vi "query.vi"(0 "object in":refnum<class "sqlite.lvclass">, 1 "database":string(combo), 2 "table输入":string(combo), 3 "columns":string[](array[string]), 4 "condition":string, 5 "error in (no error)":errorcluster) -> (14 "object out":refnum<class "sqlite.lvclass">, 15 "data":string[][](table), 16 "columns输出":string[](array[string]), 17 "拆分数据":bool, 19 "error out":errorcluster)   [LabVIEW 2016, in "sqlite.lvclass"]
uses:
  sqlite.lvclass
  <vilib>/Utility/sysdir.llb/System Directory Type.ctl
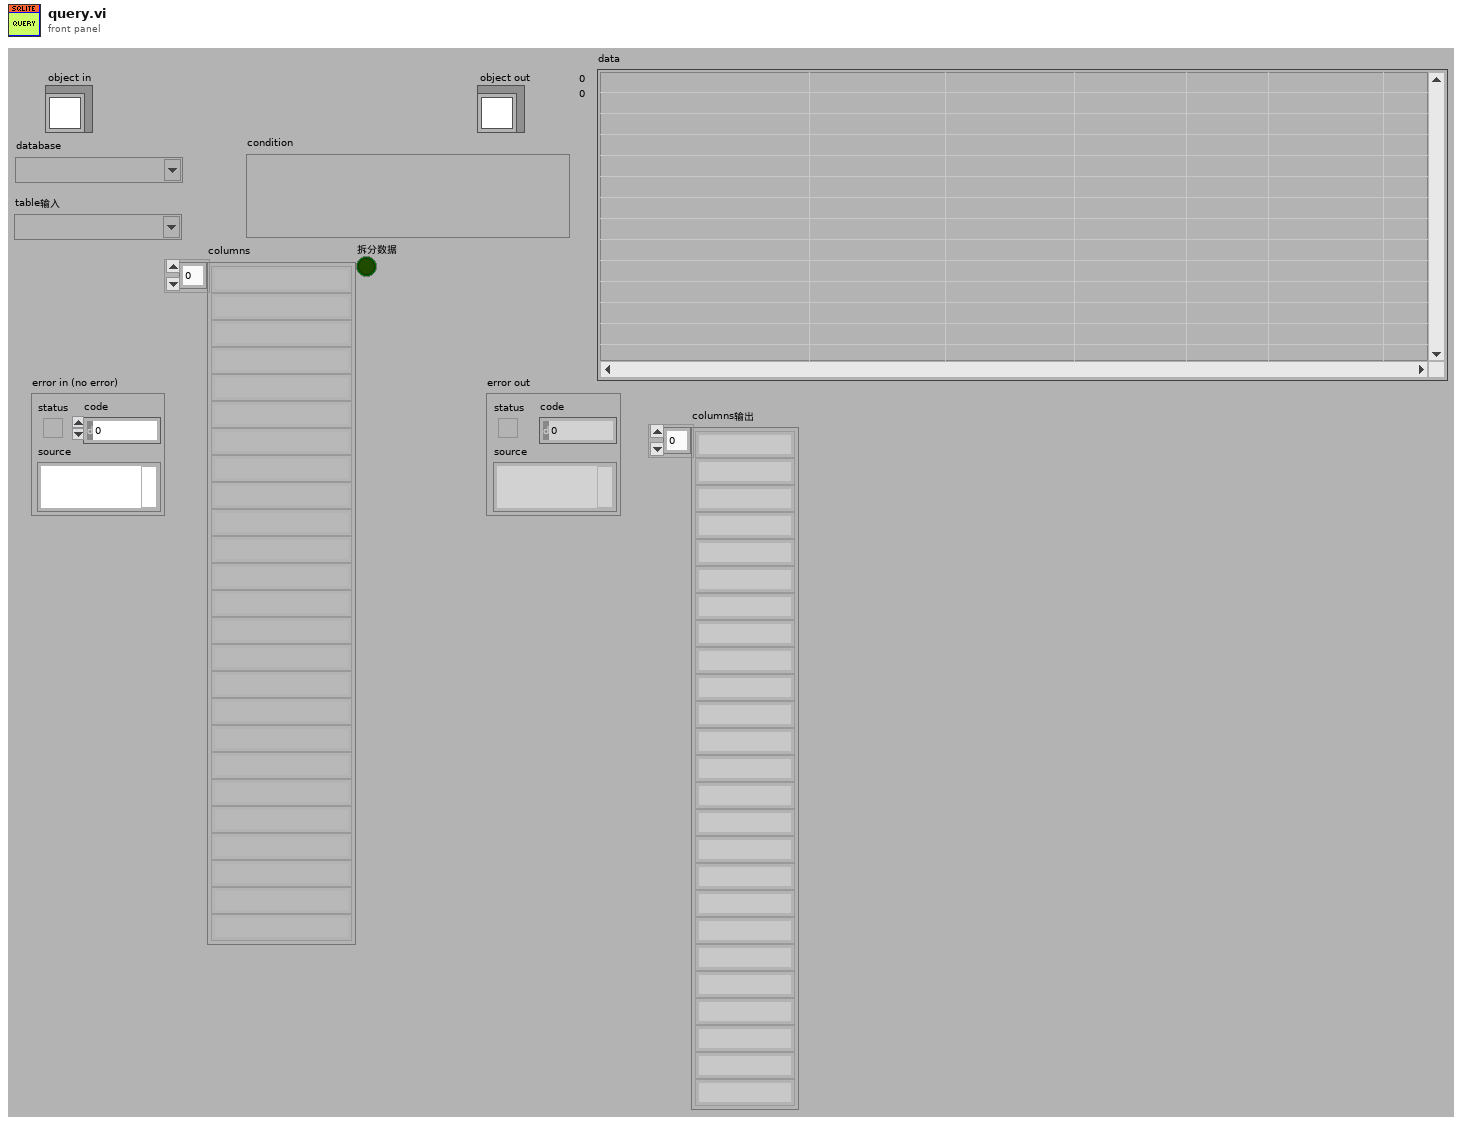
[diagram p1: front panel]
types:
  T1 = typedef "System Directory Type.ctl" = i32
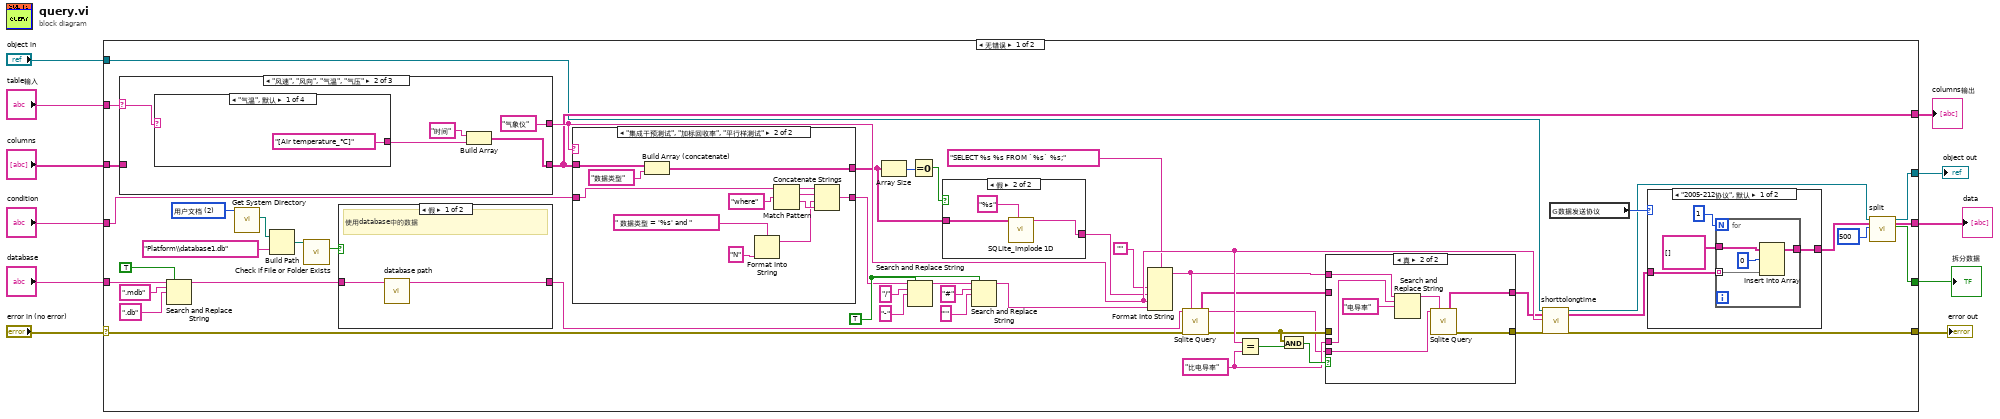
[diagram p0: block diagram]
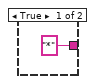
[diagram p3: hidden frame]
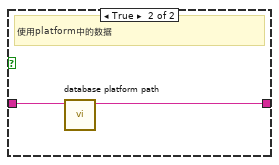
[diagram p4: hidden frame]
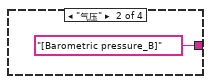
[diagram p8: hidden frame]
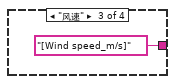
[diagram p9: hidden frame]
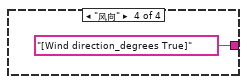
[diagram p10: hidden frame]
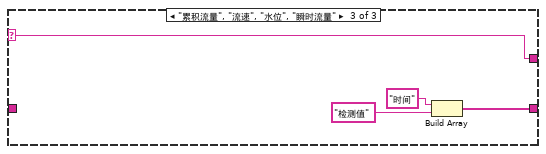
[diagram p11: hidden frame]
diagram:
  n1 = case shown="无错误" "error in (no error)" {
    selector: "error in (no error)" -> [w57 w118]
    tunnel: [w54 w118] -> w2
    tunnel: [w14 w117] -> w5
    tunnel: "object in" -> [w53 w117]
    tunnel: "table输入" -> [w61 _]
    tunnel: "columns" -> [w60 _]
    tunnel: "database" -> [w58 _]
    tunnel: [w56 _] -> w3
    tunnel: "condition" -> [w55 _]
    tunnel: [w13 _] -> w4
    tunnel: [w12 _] -> w1
    frame No Error {
      w26 = "比电导率" ("y")
      w33 = TRUE ("替换全部？(F)")
      w47 = T1 2 items=["用户目录"=0, "用户桌面"=1, "用户文档"=2, "用户应用程序数据"=3, "用户设置"=4, "用户临时目录"=5, "公共文档"=6, "公共应用程序数据"=7, "公共设置"=8, "公共缓存"=13, "系统核心库"=9, "系统安装库"=10, "应用程序文件"=11, "启动盘根目录"=12] ("system directory type")
      n2 = case shown="\"风速\", \"风向\", \"气温\", \"气压\"" w61 {
        selector: w61 -> [w103 w107 w113]
        tunnel: [w103 "气象仪" w113] -> w59
        tunnel: w60 -> [w102 _ _]
        tunnel: [w102 w104 w115] -> w56
        frame "", Default {
        }
        frame "风速", "风向", "气温", "气压" {
          n3 = case shown="\"气温\", 默认" w107 {
            tunnel: ["[Air temperature_℃]" "[Barometric pressure_B]" "[Wind speed_m/s]" "[Wind direction_degrees True]"] -> w105
            frame "气温", Default {
            }
            frame "气压" {
            }
            frame "风速" {
            }
            frame "风向" {
            }
          }
          n4 = Build Array("时间", w105) -> (w104:string[])
        }
        frame "累积流量", "流速", "水位", "瞬时流量" {
          n5 = Build Array("时间", "检测值") -> (w115:string[])
        }
      }
      n6 = Search and Replace String(replace all?=TRUE ("替换全部？(F)"), input string=w58, search string=".mdb" ("搜索字符串"), replace string=".db" ("替换字符串(\"\")")) -> (result string=w32:string)  [unwired: 4 in, 3 out]
      n7 = call <vilib>:"Get System Directory.vi"("system directory type"=w47) -> ("system directory"=w46:path)  [unwired: 10 in]
      n8 = Build Path(base path=w46, name or relative path="Platform\\database1.db" ("condition")) -> (appended path=w48:path)
      n9 = call <vilib>:"Check if File or Folder Exists.vi"("path"=w48) -> ("file or folder exists?"=w50:bool)  [unwired: 8 in, 2 out]
      n10 = case shown="假" w50 {
        tunnel: [w76 w77] -> w24
        tunnel: w32 -> [w75 w78]
        frame False {
          # "使用database中的数据"
          n11 = call "database path.vi"("database"=w75) -> ("Path out"=w76:string)  [unwired: 9 in, 1 out]
        }
        frame True {
          # "使用platform中的数据"
          n12 = call "database platform path.vi"("database"=w78) -> ("Path out"=w77:string)  [unwired: 10 in]
        }
      }
      n13 = case shown="\"集成干预测试\", \"加标回收率\", \"平行样测试\"" w59 {
        tunnel: w55 -> [w80 w85]
        tunnel: w56 -> [w79 w87]
        tunnel: [w79 w86] -> w21
        tunnel: [w80 w84] -> w20
        frame "假", Default {
        }
        frame "集成干预测试", "加标回收率", "平行样测试" {
          n14 = Build Array (concatenate)(w87, "数据类型" ("元素")) -> (w86:string[])
          n15 = Format Into String(format string=" 数据类型 = '%s' and " ("字符串"), "N" ("输入参数")) -> (resulting string=w82:string)  [unwired: 2 in, 1 out]
          n16 = Match Pattern(string=w85, regular expression="where" ("正则表达式")) -> (before substring=w90:string, match substring=w89:string, after substring=w88:string)  [unwired: 1 in, 1 out]
          n17 = Concatenate Strings(w90, w89, w82, w88) -> (w84:string)
        }
      }
      n18 = Array Size(array=w21) -> (size(s)=w45:i32)
      n19 = Search and Replace String(replace all?=w33, input string=w20, search string="/" ("搜索字符串"), replace string="-" ("替换字符串(\"\")")) -> (result string=w39:string)  [unwired: 4 in, 3 out]
      n20 = Equal To 0?(x=w45) -> (x = 0?=w44:bool)
      n21 = case shown="假" w44 {
        tunnel: w21 -> [_ w73]
        tunnel: ["*" ("t") w72] -> w42
        frame True {
        }
        frame False {
          n22 = call <userlib>:"SQLite_Implode 1D.vi"("Values"=w73, "format string"="%s") -> ("imploded string"=w72:string)  [unwired: 7 in, 1 out]
        }
      }
      n23 = Search and Replace String(replace all?=w33, input string=w39, search string="#" ("搜索字符串"), replace string="'" ("替换字符串(\"\")")) -> (result string=w22:string)  [unwired: 4 in, 3 out]
      n24 = Format Into String(format string="SELECT %s %s FROM `%s` %s;" ("SQL Query"), "", w42, w59, w22) -> (resulting string=w28:string)  [unwired: 2 in, 1 out]
      n25 = call "Sqlite Query.vi"("DB Path"=w24, "SQL Query"=w28, "error in (no error)"=w57) -> ("Results"=w29:string[][], "DB Path Out"=w25:string, "error out"=w27:errorcluster)  [unwired: 10 in]
      n26 = Equal?(x=w59, y=w26) -> (x = y?=w31:bool)
      n27 = And(x=w27, y=w31) -> (x .and. y?=w30:bool)
      n28 = case shown="真" w30 {
        tunnel: w29 -> [w63 _]
        tunnel: [w63 w70] -> w19
        tunnel: w28 -> [_ w67]
        tunnel: w25 -> [_ w69]
        tunnel: [w62 w68] -> w18
        tunnel: w27 -> [w62 _]
        tunnel: w26 -> [_ w66]
        frame False {
        }
        frame True {
          n29 = Search and Replace String(input string=w67, search string=w66, replace string="电导率" ("Tables Name")) -> (result string=w64:string)  [unwired: 5 in, 3 out]
          n30 = call "Sqlite Query.vi"("DB Path"=w69, "SQL Query"=w64) -> ("Results"=w70:string[][], "error out"=w68:errorcluster)  [unwired: 11 in, 1 out]
        }
      }
      n31 = call-dynamic "shorttolongtime.vi"("object in"=w53, "data"=w19, "table输入"=w59, "error in (no error)"=w18) -> ("object out"=w17:refnum<class "sqlite.lvclass">, "输出数组"=w51:string[][], "error out"=w54:errorcluster)  [unwired: 13 in]
      n32 = global read "断电保存全局.vi" "数据发送协议"() -> (w52:enum16{"2005-212协议", "2017-212协议"})
      n33 = case shown="\"2005-212协议\", 默认" w52 {
        tunnel: w51 -> [w94 w101]
        tunnel: [w93 w101] -> w16
        frame "2005-212协议", Default {
          n34 = for {
            N: 1 -> [_]
            tunnel: string[][] [] ("data") -> [w100]
            tunnel: w94 -> [w99] mode=indexing
            tunnel: [w97] -> w93
            n35 = Insert Into Array(array=w100, index (row)=0 ("索引 (行)"), new element=w99) -> (w97:string[][])  [unwired: 1 in]
          }
        }
        frame "2017-212协议" {
        }
      }
      n36 = call-dynamic "split.vi"("object in"=w17, "输入数据"=w16, "拆分大小"=500) -> ("object out"=w14:refnum<class "sqlite.lvclass">, "输出数组"=w13:string[][], "拆分数据"=w12:bool)  [unwired: 13 in, 1 out]
    }
    frame Error {
    }
  }
  "error out" <- w2
  "object out" <- w5
  "data" <- w4
  "columns输出" <- w3
  "拆分数据" <- w1
